vi "Session Create.vi"(8 "error in (no error)":errorcluster, 11 "ONNX Class in":refnum<class "ONNX Class.lvclass">) -> (0 "error out":errorcluster, 3 "ONNX Class out":refnum<class "ONNX Class.lvclass">)   [LabVIEW 2017, in "ONNX Class Library.lvlib" / "ONNX Class.lvclass"]
uses:
  ONNX Class.lvclass
  ONNX Class.lvclass/ONNX Class.ctl
  ONNX Class Library.lvlib
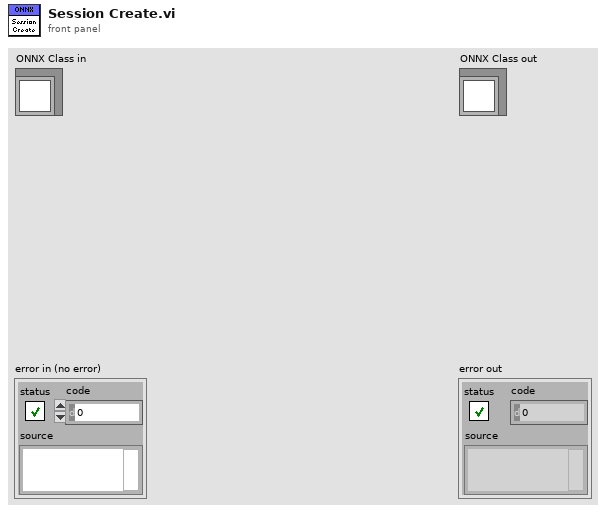
[diagram p1: front panel]
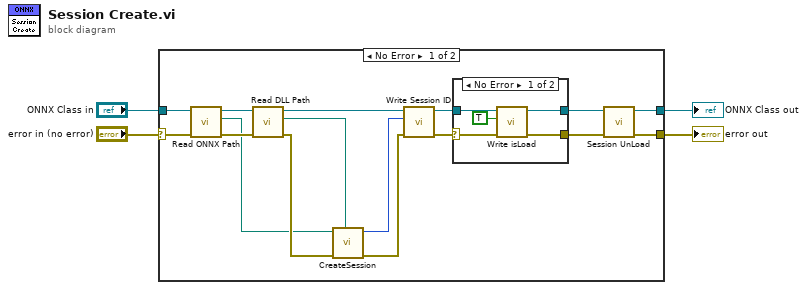
[diagram p0: block diagram]
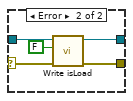
[diagram p2: hidden frame]
diagram:
  n1 = case shown="No Error" "error in (no error)" {
    selector: "error in (no error)" -> [w20 w32]
    tunnel: [w11 w32] -> w1
    tunnel: [w13 w31] -> w2
    tunnel: "ONNX Class in" -> [w18 w31]
    frame No Error {
      n2 = call-dynamic "Read ONNX Path.vi"("error in (no error)"=w20, "ONNX Class in"=w18) -> ("error out"=w9:errorcluster, "ONNX Path"=w7:path, "ONNX Class out"=w10:refnum<class "ONNX Class.lvclass">)  [unwired: 7 in]
      n3 = call-dynamic "Read DLL Path.vi"("error in (no error)"=w9, "ONNX Class in"=w10) -> ("error out"=w8:errorcluster, "DLL Path"=w6:path, "ONNX Class out"=w5:refnum<class "ONNX Class.lvclass">)  [unwired: 7 in]
      n4 = call "CreateSession.vi"("DLL path"=w6, "error in (no error)"=w8, "ONNX model path"=w7) -> ("error out"=w19:errorcluster, "session id out"=w15:i32)  [unwired: 7 in]
      n5 = call-dynamic "Write Session ID.vi"("error in (no error)"=w19, "Session ID"=w15, "ONNX Class in"=w5) -> ("error out"=w17:errorcluster, "ONNX Class out"=w16:refnum<class "ONNX Class.lvclass">)  [unwired: 7 in]
      n6 = case shown="No Error" w17 {
        selector: w17 -> [w24 w29]
        tunnel: [w22 w27] -> w12
        tunnel: w16 -> [w25 w30]
        tunnel: [w23 w28] -> w14
        frame No Error {
          n7 = call-dynamic "Write isLoad.vi"("error in (no error)"=w24, "isLoad"=TRUE, "ONNX Class in"=w25) -> ("error out"=w22:errorcluster, "ONNX Class out"=w23:refnum<class "ONNX Class.lvclass">)  [unwired: 7 in]
        }
        frame Error {
          n8 = call-dynamic "Write isLoad.vi"("error in (no error)"=w29, "isLoad"=FALSE, "ONNX Class in"=w30) -> ("error out"=w27:errorcluster, "ONNX Class out"=w28:refnum<class "ONNX Class.lvclass">)  [unwired: 7 in]
        }
      }
      n9 = call-dynamic "Session UnLoad.vi"("error in (no error)"=w12, "ONNX Class in"=w14) -> ("error out"=w11:errorcluster, "ONNX Class out"=w13:refnum<class "ONNX Class.lvclass">)  [unwired: 8 in]
    }
    frame Error {
    }
  }
  "error out" <- w1
  "ONNX Class out" <- w2
